vi "Toggle Manual Standby.vi"(8 "error in":errorcluster, 10 "Standby":bool, 11 "Launcher in":refnum<class "Launcher.lvclass">) -> (0 "error out":errorcluster, 3 "Launcher out":refnum<class "Launcher.lvclass">)   [LabVIEW 2023, in "Launcher.lvlib" / "Launcher.lvclass"]
uses:
  Library/Launcher.lvclass
  Library/Launcher.lvclass/Launcher.ctl
  builds/Base Software/Base Software.lvlibp/Base Software Messages/Respond to Menu Event Msg/Respond to Menu Event Msg.lvclass
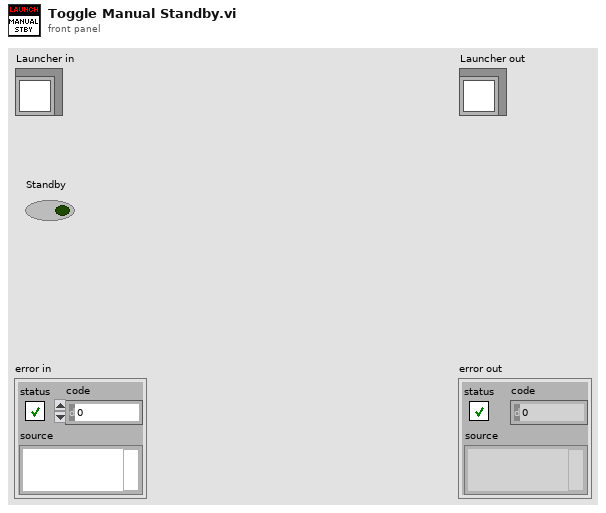
[diagram p1: front panel]
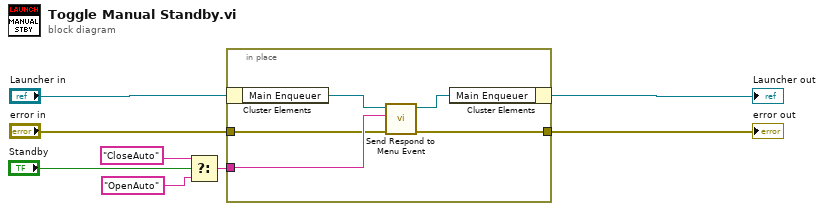
[diagram p0: block diagram]
diagram:
  n1 = Select(t="CloseAuto", s="Standby", f="OpenAuto") -> (s? t:f=w3:string)
  n2 = in-place {
    in-place-border: w3 -> [w11]
    in-place-border: "error in" -> [w10]
    in-place-border: [w9] -> w1
    n3 = in-place-cluster #1("Launcher in") -> ("Main Enqueuer"=w13:refnum<class "Message Enqueuer.lvclass">)
    n4 = call "Send Respond to Menu Event.vi"("error in (no error)"=w10, "Selection"=w11, "Message Enqueuer"=w13) -> ("error out"=w9:errorcluster, "Message Enqueuer out"=w12:refnum<class "Message Enqueuer.lvclass">)  [unwired: 7 in]
    n5 = in-place-cluster #1("Main Enqueuer"=w12) -> (→"Launcher out":refnum<class "Launcher.lvclass">)
  }
  "error out" <- w1
